vi "DBVar TimeStamp.vi"(0 "data in":variant, 2 "type":variant, 5 "initial data in":variant, 11 "error in (no error)":errorcluster, 12 "initial error in":errorcluster) -> (4 "data out":variant, 15 "error out":errorcluster)   [LabVIEW 2020, in "NI_DB Variant To Data Support.lvlib"]
uses:
  <vilib>/addons/database/_DB Variant To Data/NI_DB Variant To Data Support.lvlib
panel:
  # "terminals:\ndata in = 0\ntype = 2\ndata out = 4\ninitial data in = 5\nerror in = 11\ninitial error in = 12\nerror out = 15"
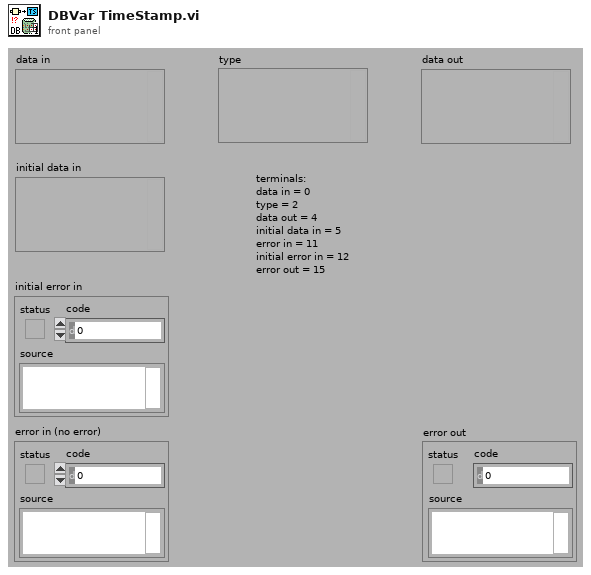
[diagram p1: front panel]
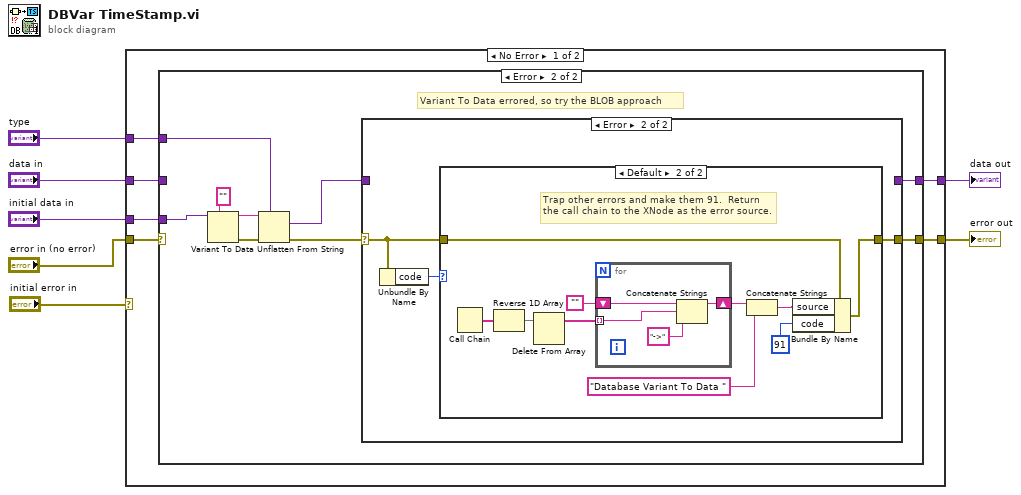
[diagram p0: block diagram]
diagram:
  n1 = case shown="No Error" "initial error in" {
    selector: "initial error in" -> [_ w45]
    tunnel: [w13 w45] -> w7
    tunnel: "data in" -> [w11 w44]
    tunnel: [w12 w44] -> w6
    tunnel: "error in (no error)" -> [w10 _]
    tunnel: "type" -> [w9 _]
    tunnel: "initial data in" -> [w8 _]
    frame No Error {
      n2 = case shown="Error" w10 {
        selector: w10 -> [w14 _]
        tunnel: [w14 w24] -> w13
        tunnel: [w15 w23] -> w12
        tunnel: w11 -> [w15 _]
        tunnel: w9 -> [_ w18]
        tunnel: w8 -> [_ w17]
        frame No Error {
          # "Variant To Data succeeded"
        }
        frame Error {
          # "Variant To Data errored, so try the BLOB approach"
          n3 = Variant To Data(type="", Variant=w17) -> (data=w21:string, error out=w20:errorcluster)  [unwired: 1 in]
          n4 = Unflatten From String(type=w18, binary string=w21, error in (no error)=w20) -> (value=w16:variant, error out=w19:errorcluster)  [unwired: 2 in, 1 out]
          n5 = case shown="Error" w19 {
            selector: w19 -> [w25 w27]
            tunnel: [w25 w29] -> w24
            tunnel: [w26 _] -> w23
            tunnel: w16 -> [w26 _]
            frame No Error {
              # "pass through warnings"
            }
            frame Error {
              n6 = Unbundle By Name(w27) -> ("code"=w28:i32)
              n7 = case shown="Default" w28 {
                tunnel: [_ w39] -> w29
                tunnel: w27 -> [_ w30]
                frame -2147467261 {
                  # "Variant To Data returns -2147467261 if the variant input is NULL.  We want to clear the error and pass back default data."
                }
                frame Default {
                  # "Trap other errors and make them 91.  Return the call chain to the XNode as the error source."
                  n8 = Call Chain() -> (call chain=w36:string[])
                  n9 = Reverse 1D Array(array=w36) -> (reversed array=w35:string[])
                  n10 = Delete From Array(array=w35) -> (array with subset deleted=w34:string[])  [unwired: 2 in, 1 out]
                  n11 = for {
                    tunnel: w34 -> [w42] mode=indexing
                    shift-right: [w43] -> w33
                    shift-left: "" -> [w41]
                    n12 = Concatenate Strings(w41, w42, "->" ("string")) -> (w43:string)
                  }
                  n13 = Concatenate Strings(w33, "Database Variant To Data " ("source")) -> (w37:string)
                  n14 = Bundle By Name(cluster=w30, "source"=w37, "code"=91) -> (w39:errorcluster)
                }
              }
            }
          }
        }
      }
    }
    frame Error {
      # "keep previous error if one occurred"
    }
  }
  "error out" <- w7
  "data out" <- w6
